vi "AI Reg UI.vi"(8 "error in (no error)":errorcluster, 11 "Node Ptr":T3 format="%.0x") -> (0 "error out":errorcluster)   [LabVIEW 2015, in "Modbus Master System Explorer.lvlib"]
uses:
  Modbus Master System Explorer.lvlib
  <vilib>/NI Veristand/Custom Device API/Custom Device Item Ref.ctl
  Shared/Controls/Data Model/DataType.ctl
  SubVIs/Radix.ctl
  <vilib>/NI VeriStand/Custom Device API/Custom Device API.lvlib
  Shared/Modbus Master Shared.lvlib
panel:
  in  "Radix":T1
  out "Registers":i32
  in  "DataType":T2
  in  "Sub-Index (Bool)":u16
  in  "Valid?":string
  in  "Address":u16
  in  "Header":cluster{"Section Name":string}={"Section Name"="Input Register (Analog Input) Settings"}
  in  "Description":string
  in  "Name":string
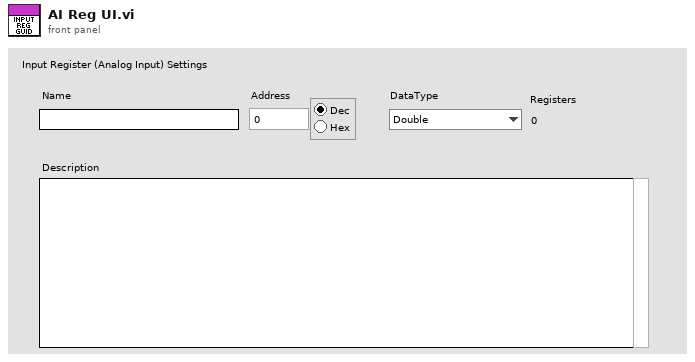
[diagram p1: front panel]
types:
  T1 = typedef "Modbus Master System Explorer.lvlib/Radix.ctl" = enum32{"Decimal", "Hexidecimal"}
  T2 = typedef "Modbus Master Shared.lvlib/DataType.ctl" = enum16{"Double", "Single", "I64", "I32", "I16", "I8", "U64", "U32", "U16", "U8", "Boolean"}
  T3 = typedef "Custom Device API.lvlib/Custom Device Item Ref.ctl" = u64
  T4 = typedef "Custom Device API.lvlib/Custom Device Commands.ctl" = enum16{"Default", "Item renamed", "Shutdown", "Dynamic button pressed"}
  T5 = typedef "Custom Device API.lvlib/Custom Device Item Info.ctl" = cluster{"Name":string, "Is Channel":bool, "GUID":string, "Is Waveform":bool}
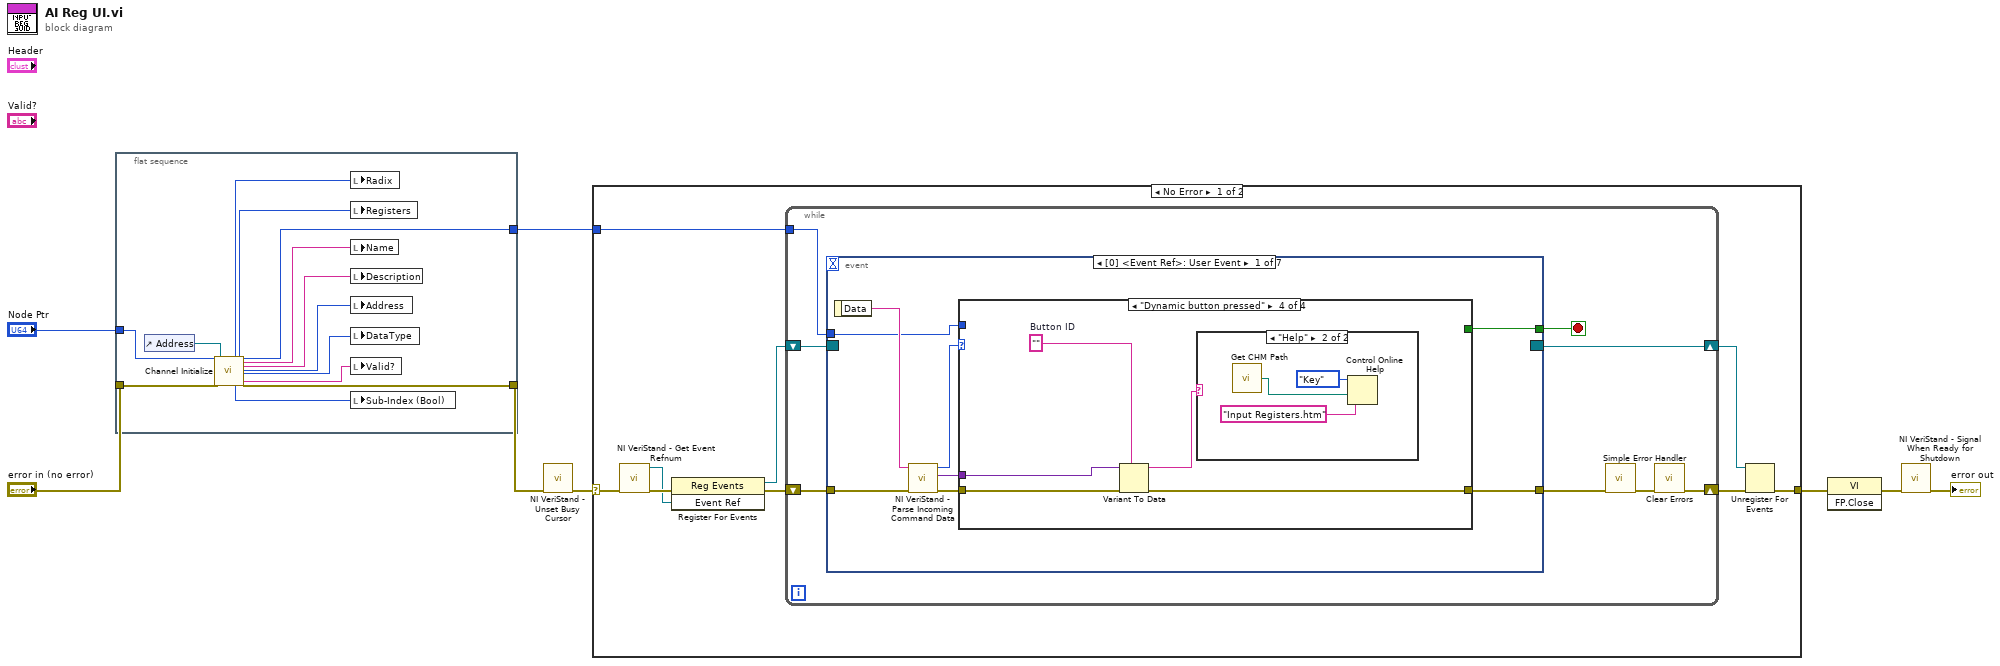
[diagram p0: block diagram]
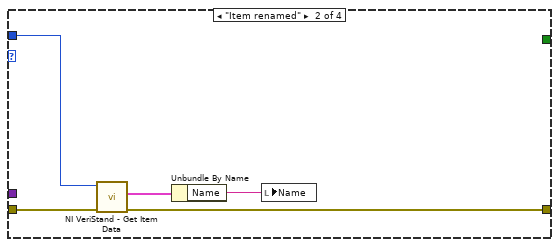
[diagram p3: hidden frame]
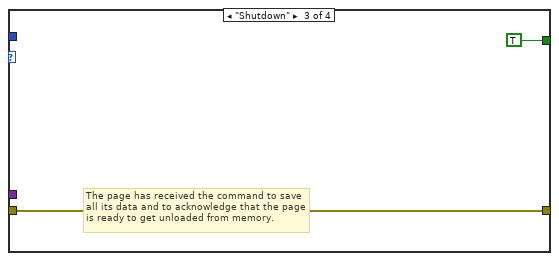
[diagram p4: hidden frame]
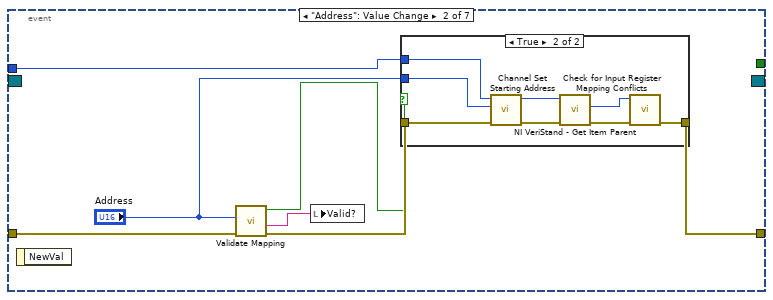
[diagram p6: hidden frame]
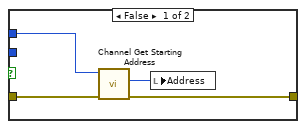
[diagram p7: hidden frame]
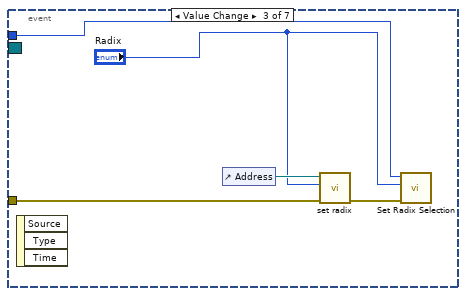
[diagram p8: hidden frame]
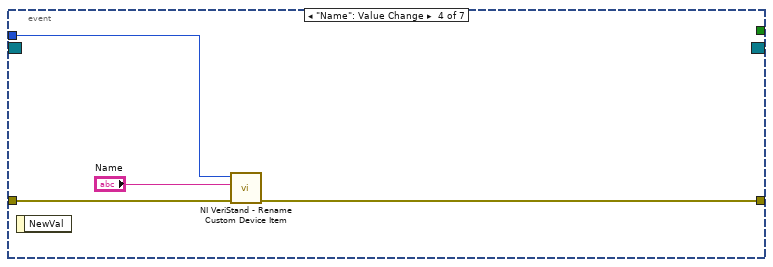
[diagram p9: hidden frame]
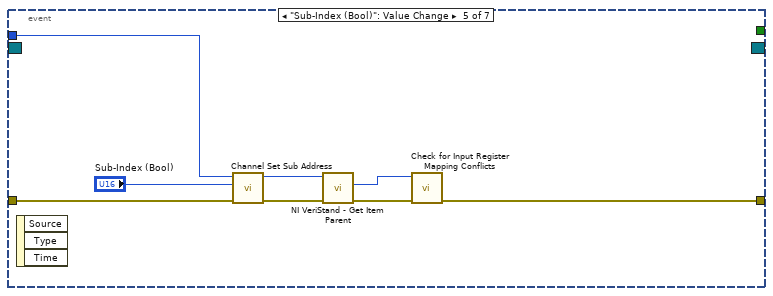
[diagram p10: hidden frame]
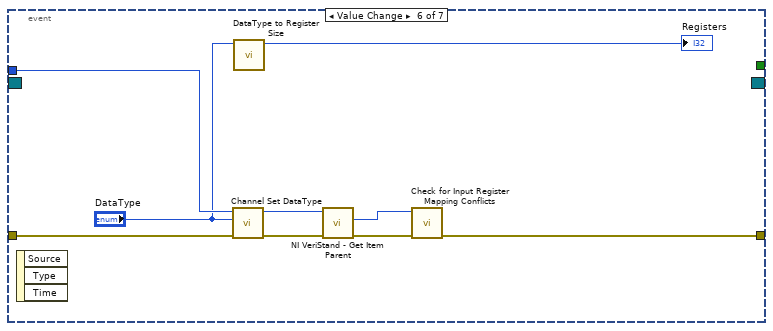
[diagram p11: hidden frame]
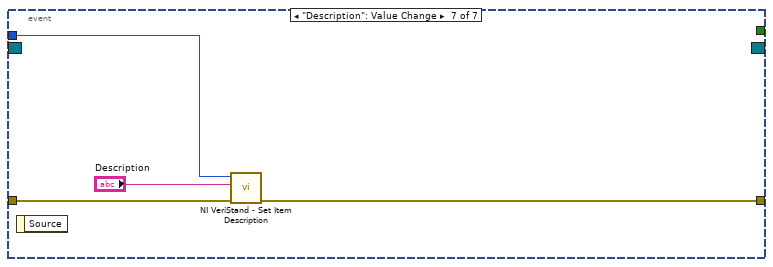
[diagram p12: hidden frame]
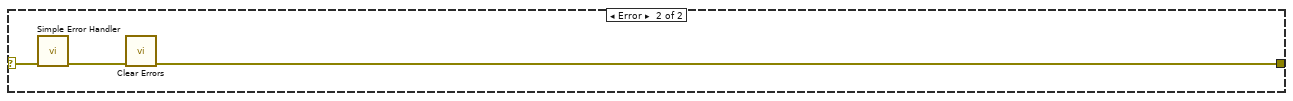
[diagram p13: hidden frame]
diagram:
  n1 = flat-sequence {
    tunnel: "Node Ptr" -> [w12]
    tunnel: [w11] -> w3
    tunnel: "error in (no error)" -> [w10]
    tunnel: [w9] -> w1
    frame #0 {
      n2 = control-ref of="Address"() -> (w13:refnum<vi>)
      n3 = call "Channel Initialize.vi"("Item Ref in"=w12, "error in (no error)"=w10, "Starting Address Ref in"=w13) -> ("Radix"=w15:T1, "Sub-Index (Bool)"=w16:u16, "Registers"=w17:i32, "Channel Ref out"=w11:T3, "Name"=w20:string, "Description"=w21:string, "Starting Address"=w18:u16, "DataType"=w19:T2, "Status Message"=w14:string, "error out"=w9:errorcluster)  [unwired: 13 in, 2 out]
      n4 = local write "Radix"(w15) -> ()
      n5 = local write "Registers"(w17) -> ()
      n6 = local write "Name"(w20) -> ()
      n7 = local write "Description"(w21) -> ()
      n8 = local write "Address"(w18) -> ()
      n9 = local write "DataType"(w19) -> ()
      n10 = local write "Valid?"(w14) -> ()
      n11 = local write "Sub-Index (Bool)"(w16) -> ()
    }
  }
  n12 = call <vilib>:"NI VeriStand - Unset Busy Cursor.vi"("error in (no error)"=w1) -> ("error out"=w5:errorcluster)  [unwired: 10 out]
  n13 = case shown="No Error" w5 {
    selector: w5 -> [w22 w114]
    tunnel: [w27 w112] -> w8
    tunnel: w3 -> [w23 _]
    frame No Error {
      n14 = call <vilib>:"NI VeriStand - Get Event Refnum.vi"("error in (no error)"=w22) -> ("error out"=w30:errorcluster, "Event Ref"=w26:refnum<user-event>)  [unwired: 9 out]
      n15 = register-events(error in=w30, w26) -> (reference out=w24:refnum<event-registration>, error out=w25:errorcluster)  [unwired: 1 in]
      n16 = while {
        tunnel: w23 -> [w34]
        shift-right: [w31] -> w28
        shift-left: w25 -> [w37]
        shift-right: [w38] -> w29
        shift-left: w24 -> [w36]
        stop <- w35 stop-if-true
        n17 = event shown="[0] <Event Ref>: User Event" {
          selector: w36 -> [_ _ _ _ _ _ _]
          dyn-events: [_ _ _ _ _ _ _] -> w38
          timeout: _ -> [_ _ _ _ _ _ _]
          tunnel: w37 -> [w46 w67 w85 w90 w96 w106 w110]
          tunnel: [w42 _ _ _ _ _ _] -> w35
          tunnel: [w41 w68 _ w89 w92 w101 w109] -> w33
          tunnel: w34 -> [w40 w69 w84 w88 w97 w107 w111]
          event User Event {
            n18 = event-data() -> ("Data"=w45:string)  [unwired: 1 out]
            n19 = call <vilib>:"NI VeriStand - Parse Incoming Command Data.vi"("error in (no error)"=w46, "Incoming data"=w45) -> ("error out"=w44:errorcluster, "Outgoing data"=w39:variant, "Action"=w43:T4)  [unwired: 7 out]
            n20 = case shown="\"Dynamic button pressed\"" w43 {
              tunnel: w44 -> [w47 w52 w53 w59]
              tunnel: [_ _ TRUE _] -> w42
              tunnel: [w47 w49 w53 w56] -> w41
              tunnel: w40 -> [_ w51 _ _]
              tunnel: w39 -> [_ _ _ w58]
              frame "Default", Default {
              }
              frame "Item renamed" {
                n21 = call <vilib>:"NI VeriStand - Get Item Data.vi"("error in (no error)"=w52, "Item Ref in"=w51) -> ("error out"=w49:errorcluster, "Item Info"=w50:T5)  [unwired: 8 out]
                n22 = Unbundle By Name(w50) -> ("Name"=w48:string)
                n23 = local write "Name"(w48) -> ()
              }
              frame "Shutdown" {
                # "The page has received the command to save all its data and to acknowledge that the page is ready to get unloaded from memory."
              }
              frame "Dynamic button pressed" {
                w57 = ""  # Button ID
                n24 = Variant To Data(error in=w59, type=w57, Variant=w58) -> (data=w55:string, error out=w56:errorcluster)
                n25 = case shown="\"Help\"" w55 {
                  frame Default {
                  }
                  frame "Help" {
                    n26 = call "Get CHM Path.vi"() -> ("appended path"=w62:path)
                    n27 = Control Online Help(2:w62, 3:"Input Registers.htm" ("String to search for"), 4:enum16{"Contents", "Key", "Close"}."Key" ("Operation")) -> ()  [unwired: 1 in, 1 out]
                  }
                }
              }
            }
          }
          event "Address": Value Change {
            n28 = event-data() -> ()  [unwired: 2 out]
            n29 = call "Validate Mapping.vi"("error in (no error)"=w67, "Mapping"="Address") -> ("error out"=w66:errorcluster, "Status Message"=w65:string, "Valid?"=w64:bool)  [unwired: 7 in]
            n30 = local write "Valid?"(w65) -> ()
            n31 = case shown="True" w64 {
              tunnel: w69 -> [w73 w80]
              tunnel: [w70 w75] -> w68
              tunnel: w66 -> [w71 w81]
              tunnel: "Address" -> [_ w79]
              frame False {
                n32 = call "Channel Get Starting Address.vi"("error in (no error)"=w71, "Item Ref in"=w73) -> ("error out"=w70:errorcluster, "Value"=w72:u16)  [unwired: 7 in, 1 out]
                n33 = local write "Address"(w72) -> ()
              }
              frame True {
                n34 = call "Channel Set Starting Address.vi"("error in (no error)"=w81, "Value"=w79, "Item Ref in"=w80) -> ("error out"=w78:errorcluster, "Item Ref out"=w77:T3)  [unwired: 7 in]
                n35 = call <vilib>:"NI VeriStand - Get Item Parent.vi"("error in (no error)"=w78, "Item Ref in"=w77) -> ("error out"=w76:errorcluster, "Parent Ref"=w74:T3)  [unwired: 6 in, 2 out]
                n36 = call "Check for Input Register Mapping Conflicts.vi"("error in (no error)"=w76, "Group Ref in"=w74) -> ("error out"=w75:errorcluster)  [unwired: 6 in, 3 out]
              }
            }
          }
          event Value Change {
            n37 = event-data() -> ()  [unwired: 4 out]
            n38 = control-ref of="Address"() -> (w86:refnum<vi>)
            n39 = call "set radix.vi"("error in (no error)"=w85, "Radix"="Radix", "Digital in"=w86) -> ("error out"=w82:errorcluster)  [unwired: 8 in]
            n40 = call "Set Radix Selection.vi"("error in (no error)"=w82, "Radix"="Radix", "Item Ref in"=w84) -> ()  [unwired: 7 in, 2 out]
          }
          event "Name": Value Change {
            n41 = event-data() -> ()  [unwired: 2 out]
            n42 = call <vilib>:"NI VeriStand - Rename Custom Device Item.vi"("error in (no error)"=w90, "New Name"="Name", "Item Ref in"=w88) -> ("error out"=w89:errorcluster)  [unwired: 1 in, 7 out]
          }
          event "Sub-Index (Bool)": Value Change {
            n43 = event-data() -> ()  [unwired: 4 out]
            n44 = call "Channel Set Sub Address.vi"("error in (no error)"=w96, "Value"="Sub-Index (Bool)", "Item Ref in"=w97) -> ("error out"=w93:errorcluster, "Item Ref out"=w91:T3)  [unwired: 7 in]
            n45 = call <vilib>:"NI VeriStand - Get Item Parent.vi"("error in (no error)"=w93, "Item Ref in"=w91) -> ("error out"=w94:errorcluster, "Parent Ref"=w95:T3)  [unwired: 6 in, 2 out]
            n46 = call "Check for Input Register Mapping Conflicts.vi"("error in (no error)"=w94, "Group Ref in"=w95) -> ("error out"=w92:errorcluster)  [unwired: 6 in, 3 out]
          }
          event Value Change {
            n47 = event-data() -> ()  [unwired: 4 out]
            n48 = call "Channel Set DataType.vi"("error in (no error)"=w106, "DataType"="DataType", "Item Ref in"=w107) -> ("error out"=w103:errorcluster, "Item Ref out"=w105:T3)  [unwired: 7 in]
            n49 = call "DataType to Register Size.vi"("DataType"="DataType") -> ("Registers"=→"Registers":i32)  [unwired: 9 in, 1 out]
            n50 = call <vilib>:"NI VeriStand - Get Item Parent.vi"("error in (no error)"=w103, "Item Ref in"=w105) -> ("error out"=w102:errorcluster, "Parent Ref"=w104:T3)  [unwired: 6 in, 2 out]
            n51 = call "Check for Input Register Mapping Conflicts.vi"("error in (no error)"=w102, "Group Ref in"=w104) -> ("error out"=w101:errorcluster)  [unwired: 6 in, 3 out]
          }
          event "Description": Value Change {
            n52 = event-data() -> ()  [unwired: 2 out]
            n53 = call <vilib>:"NI VeriStand - Set Item Description.vi"("error in (no error)"=w110, "Description"="Description", "Item Ref in"=w111) -> ("error out"=w109:errorcluster)  [unwired: 8 out]
          }
        }
        n54 = call <vilib>:"Simple Error Handler.vi"("error in (no error)"=w33) -> ("error out"=w32:errorcluster)  [unwired: 1 in, 7 out]
        n55 = call <vilib>:"Clear Errors.vi"("error in (no error)"=w32) -> ("error out"=w31:errorcluster)  [unwired: 1 in, 5 out]
      }
      n56 = Unregister For Events(event registration refnum=w29, error in=w28) -> (error out=w27:errorcluster)
    }
    frame Error {
      n57 = call <vilib>:"Simple Error Handler.vi"("error in (no error)"=w114) -> ("error out"=w113:errorcluster)  [unwired: 1 in, 7 out]
      n58 = call <vilib>:"Clear Errors.vi"("error in (no error)"=w113) -> ("error out"=w112:errorcluster)  [unwired: 1 in, 5 out]
    }
  }
  n59 = invoke class="VI" method="FP.Close"(error in=w8) -> (error out=w7:errorcluster)  [unwired: 2 in, 2 out]
  n60 = call <vilib>:"NI VeriStand - Signal When Ready for Shutdown.vi"("error in (no error)"=w7) -> ("error out"=→"error out":errorcluster)  [unwired: 10 out]
